vi "Initialize.vi"(8 "error in (no error)":errorcluster, 11 "Bronkhorst Settings in":T1={"VISA resource name"="", "Simulated?"=FALSE, "Smoothing Steps"=1} {"Smoothing Steps" min=1 step=1}) -> (0 "error out":errorcluster, 2 "No Meter Connected":bool, 3 "Bronkhorst Settings out":T1={"VISA resource name"="", "Simulated?"=FALSE, "Smoothing Steps"=1} {"Smoothing Steps" min=1 step=1})   [LabVIEW 2021, in "Bronkhorst M14 Flow Meter.lvlib"]
uses:
  Bronkhorst M14 Flow Meter.lvlib
  Settings Cluster.ctl
  <vilib>/Instr/_visa.llb/VISA Configure Serial Port (Instr).vi
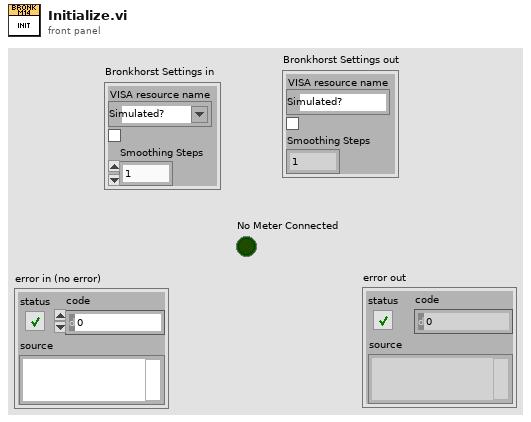
[diagram p1: front panel]
types:
  T1 = typedef "Bronkhorst M14 Flow Meter.lvlib/Settings Cluster.ctl" = cluster{"VISA resource name":refnum<visa-resource-name>, "Simulated?":bool, "Smoothing Steps":i32}
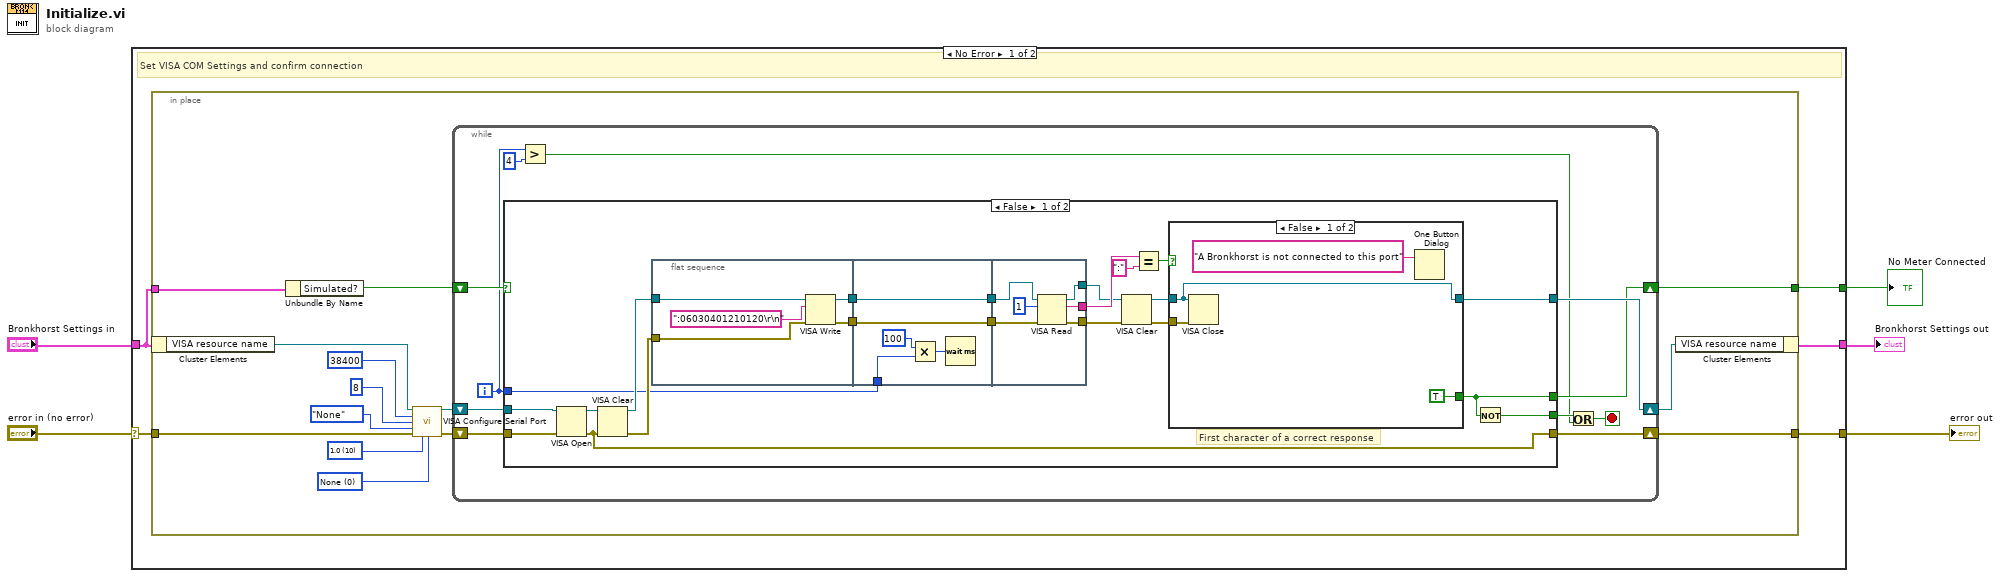
[diagram p0: block diagram]
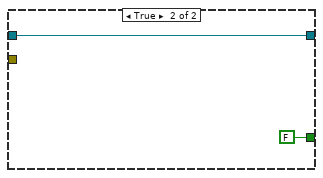
[diagram p2: hidden frame]
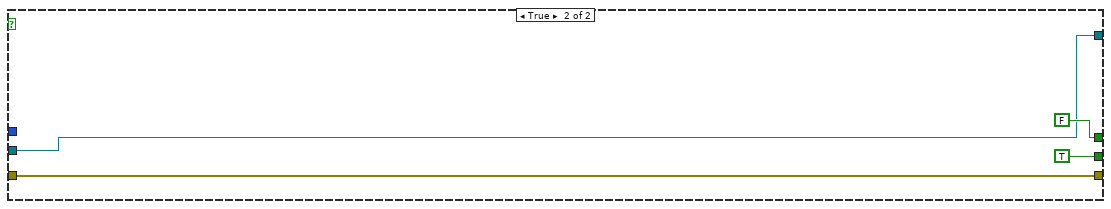
[diagram p3: hidden frame]
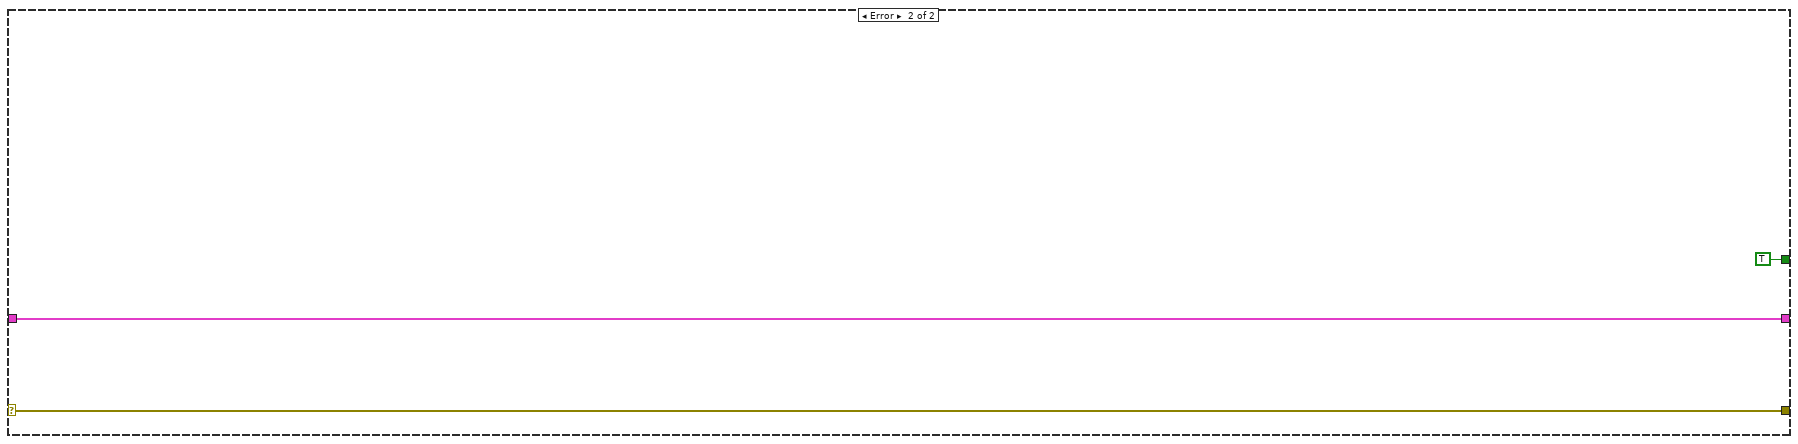
[diagram p4: hidden frame]
diagram:
  n1 = case shown="No Error" "error in (no error)" {
    selector: "error in (no error)" -> [w10 w85]
    tunnel: "Bronkhorst Settings in" -> [w8 w84]
    tunnel: [w9 w85] -> w4
    tunnel: [w7 w84] -> w2
    tunnel: [w6 TRUE] -> w1
    frame No Error {
      # "Set VISA COM Settings and confirm connection"
      n2 = in-place {
        in-place-border: w10 -> [w24]
        in-place-border: w8 -> [w22]
        in-place-border: [w21] -> w9
        in-place-border: [w18] -> w6
        w13 = u16 0 items=["None", "XON/XOFF", "RTS/CTS", "XON/XOFF & RTS/CTS", "DTR/DSR", "XON/XOFF & DTR/DSR"] ("flow control (0:none)")
        w14 = u16 10 items=["1.0"=10, "1.5"=15, "2.0"=20] ("stop bits (10: 1 bit)")
        n3 = in-place-cluster #1(w8) -> ("VISA resource name"=w20:refnum<visa-resource-name>)
        n4 = Unbundle By Name(w22) -> ("Simulated?"=w23:bool)
        n5 = call-poly "VISA Configure Serial Port"("VISA resource name"=w20, "baud rate (9600)"=u32 38400, "data bits (8)"=u16 8, "parity (0:none)"=enum16{"None", "Odd", "Even", "Mark", "Space"}."None", "error in (no error)"=w24, "stop bits (10: 1 bit)"=w14, "flow control (0:none)"=w13) -> ("VISA resource name out"=w12:refnum<visa-resource-name>, "error out"=w11:errorcluster)  [unwired: 7 in]
        n6 = while {
          shift-right: [w32] -> w18
          shift-left: w23 -> [w35]
          shift-right: [w33] -> w19
          shift-left: w12 -> [w31]
          shift-right: [w34] -> w21
          shift-left: w11 -> [w30]
          i -> [w28]
          stop <- w25 stop-if-true
          n7 = case shown="False" w35 {
            tunnel: [w56 w81] -> w34
            tunnel: [w44 w80] -> w33
            tunnel: [w37 FALSE] -> w32
            tunnel: w31 -> [w40 w80]
            tunnel: w30 -> [w39 w81]
            tunnel: w28 -> [w38 _]
            tunnel: [w36 TRUE] -> w27
            frame False {
              # "First character of a correct response"
              n8 = VISA Open(error in (no error)=w39, VISA resource name=w40) -> (VISA resource name=w41:refnum<visa-resource-name>, error out=w56:errorcluster)  [unwired: 3 in]
              n9 = VISA Clear(VISA resource name=w41, error in (no error)=w56) -> (VISA resource name out=w42:refnum<visa-resource-name>, error out=w43:errorcluster)
              n10 = flat-sequence {
                tunnel: w43 -> [w61]
                tunnel: [w59] -> w55
                tunnel: [w58] -> w54
                tunnel: w42 -> [w57]
                tunnel: w55 -> [w66]
                tunnel: [w66] -> w53
                tunnel: w54 -> [w65]
                tunnel: [w65] -> w52
                tunnel: w38 -> [w62]
                tunnel: [w72] -> w46
                tunnel: [w71] -> w50
                tunnel: [w70] -> w45
                tunnel: w53 -> [w69]
                tunnel: w52 -> [w68]
                frame #0 {
                  n11 = VISA Write(VISA resource name=w57, write buffer=":06030401210120\r\n", error in (no error)=w61) -> (VISA resource name out=w59:refnum<visa-resource-name>, error out=w58:errorcluster)  [unwired: 1 out]
                }
                frame #1 {
                  n12 = Multiply(x=u32 100 ("milliseconds to wait"), y=w62) -> (x*y=w63:u32)
                  n13 = Wait (ms)(milliseconds to wait=w63) -> ()  [unwired: 1 out]
                }
                frame #2 {
                  n14 = VISA Read(VISA resource name=w69, byte count=u32 1, error in (no error)=w68) -> (VISA resource name out=w70:refnum<visa-resource-name>, read buffer=w71:string, error out=w72:errorcluster)  [unwired: 1 out]
                }
              }
              n15 = VISA Clear(VISA resource name=w45, error in (no error)=w46) -> (VISA resource name out=w47:refnum<visa-resource-name>, error out=w48:errorcluster)
              n16 = Equal?(x=w50, y=":") -> (x = y?=w51:bool)
              n17 = case shown="False" w51 {
                tunnel: w47 -> [w74 w78]
                tunnel: w48 -> [w75 _]
                tunnel: [w74 w78] -> w44
                tunnel: [TRUE FALSE] -> w37
                frame False {
                  n18 = VISA Close(VISA resource name=w74, error in (no error)=w75) -> ()  [unwired: 1 out]
                  n19 = One Button Dialog(message="A Bronkhorst is not connected to this port") -> ()  [unwired: 1 in, 1 out]
                }
                frame True {
                }
              }
              n20 = Not(x=w37) -> (.not. x?=w36:bool)
            }
            frame True {
            }
          }
          n21 = Greater?(x=w28, y=4) -> (0:w26:bool)
          n22 = Or(x=w27, y=w26) -> (x .or. y?=w25:bool)
        }
        n23 = in-place-cluster #1("VISA resource name"=w19) -> (w7:T1)
      }
    }
    frame Error {
    }
  }
  "error out" <- w4
  "Bronkhorst Settings out" <- w2
  "No Meter Connected" <- w1
